vi "mg3694b_SetFreqPowerMod.vi"(0 "GPIB Address":string="18", 1 "Frequency (GHz)":dbl, 2 "Power (dBm)":dbl) -> ()   [LabVIEW 2014]
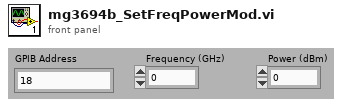
[diagram p1: front panel]
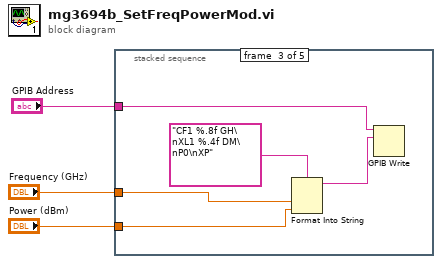
[diagram p0: block diagram]
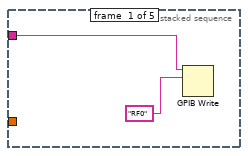
[diagram p2: hidden frame]
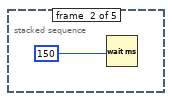
[diagram p3: hidden frame]
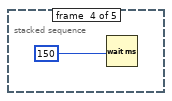
[diagram p4: hidden frame]
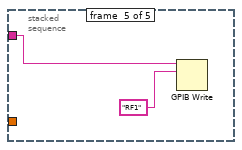
[diagram p5: hidden frame]
diagram:
  n1 = stacked-sequence {
    tunnel: "GPIB Address" -> [w4 _ w9 _ w14]
    tunnel: "Frequency (GHz)" -> [_ _ w7 _ _]
    tunnel: "Power (dBm)" -> [_ _ w8 _ _]
    frame #0 {
      n2 = GPIB Write(0:w4, 1:"RF0") -> ()  [unwired: 1 in, 4 out]
    }
    frame #1 {
      n3 = Wait (ms)(milliseconds to wait=150) -> ()  [unwired: 1 out]
    }
    frame #2 {
      n4 = Format Into String(format string="CF1 %.8f GH\nXL1 %.4f DM\nP0\nXP", w7, w8) -> (resulting string=w11:string)  [unwired: 2 in, 1 out]
      n5 = GPIB Write(0:w9, 1:w11) -> ()  [unwired: 1 in, 4 out]
    }
    frame #3 {
      n6 = Wait (ms)(milliseconds to wait=150) -> ()  [unwired: 1 out]
    }
    frame #4 {
      n7 = GPIB Write(0:w14, 1:"RF1") -> ()  [unwired: 1 in, 4 out]
    }
  }
